vi "App Config (FGV).vi"(7 "Action (Read)":T1, 8 "error in (no error)":errorcluster, 11 "DVR In":refnum<data-value>) -> (0 "error out":errorcluster, 3 "DVR Out":refnum<data-value>)   [LabVIEW 2015, in "App Config.lvlib"]
uses:
  App Config.lvlib
  FGV Action.ctl
  App Config Data.ctl
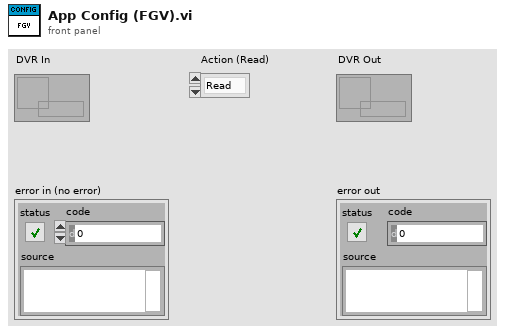
[diagram p1: front panel]
types:
  T1 = typedef "App Config.lvlib/FGV Action.ctl" = enum16{"Read", "Write"}
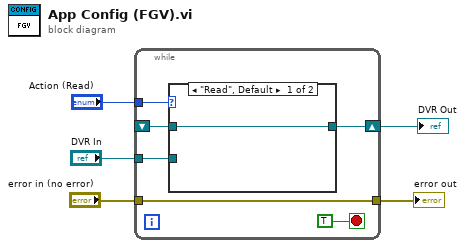
[diagram p0: block diagram]
diagram:
  n1 = while {
    tunnel: "error in (no error)" -> [w9]
    tunnel: "Action (Read)" -> [w10]
    tunnel: [w9] -> w3
    shift-right: [w7] -> w1
    shift-left: _ -> [w8]
    tunnel: "DVR In" -> [w6]
    stop <- TRUE stop-if-true
    n2 = case shown="\"Read\", Default" w10 {
      tunnel: w8 -> [w12 _]
      tunnel: [w12 w13] -> w7
      tunnel: w6 -> [_ w13]
      frame "Read", Default {
      }
      frame "Write" {
      }
    }
  }
  "error out" <- w3
  "DVR Out" <- w1
